vi "sortData.vi"(8 "error in (no error)":errorcluster, 9 "data":T1(array[cluster])=[[{"time"=0.0, "Channel"=refnum, "data"=0.8}, {"time"=29.998, "Channel"=refnum, "data"=0.0}], [{"time"=0.0, "Channel"=refnum, "data"=0.74}, {"time"=29.998, "Channel"=refnum, "data"=0.0}], [{"time"=29.998, "Channel"=refnum, "data"=0.8}, {"time"=33.5, "Channel"=refnum, "data"=0.0}]], 10 "times":dbl[](array[numeric]), 11 "ScriptEventList in":refnum<class "ScriptEventList.lvclass">) -> (0 "error out":errorcluster, 2 "data out":T1(array[cluster]), 3 "ScriptEventList out":refnum<class "ScriptEventList.lvclass">)   [LabVIEW 2011, in "Tools.lvlib" / "Scripting.lvlib" / "ScriptEventList.lvclass"]
uses:
  ScriptEventList.lvclass
  DatabaseHelpers/Database Objects/Channel/Channel.lvclass
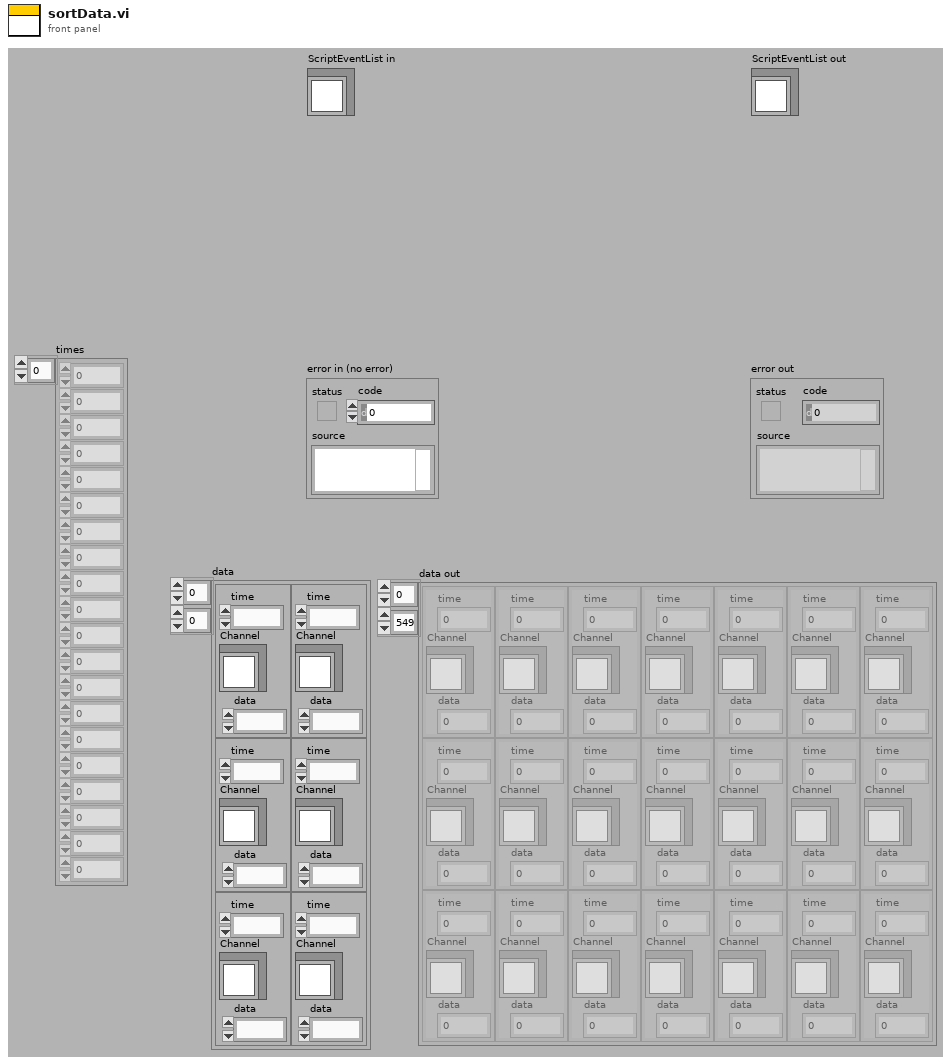
[diagram p1: front panel]
types:
  T1 = cluster{"time":dbl, "Channel":refnum<class "Channel.lvclass">, "data":dbl}[][]
  T2 = cluster{"time":dbl, "Channel":refnum<class "Channel.lvclass">, "data":dbl}[]
  T3 = cluster{"time":dbl, "Channel":refnum<class "Channel.lvclass">, "data":dbl}
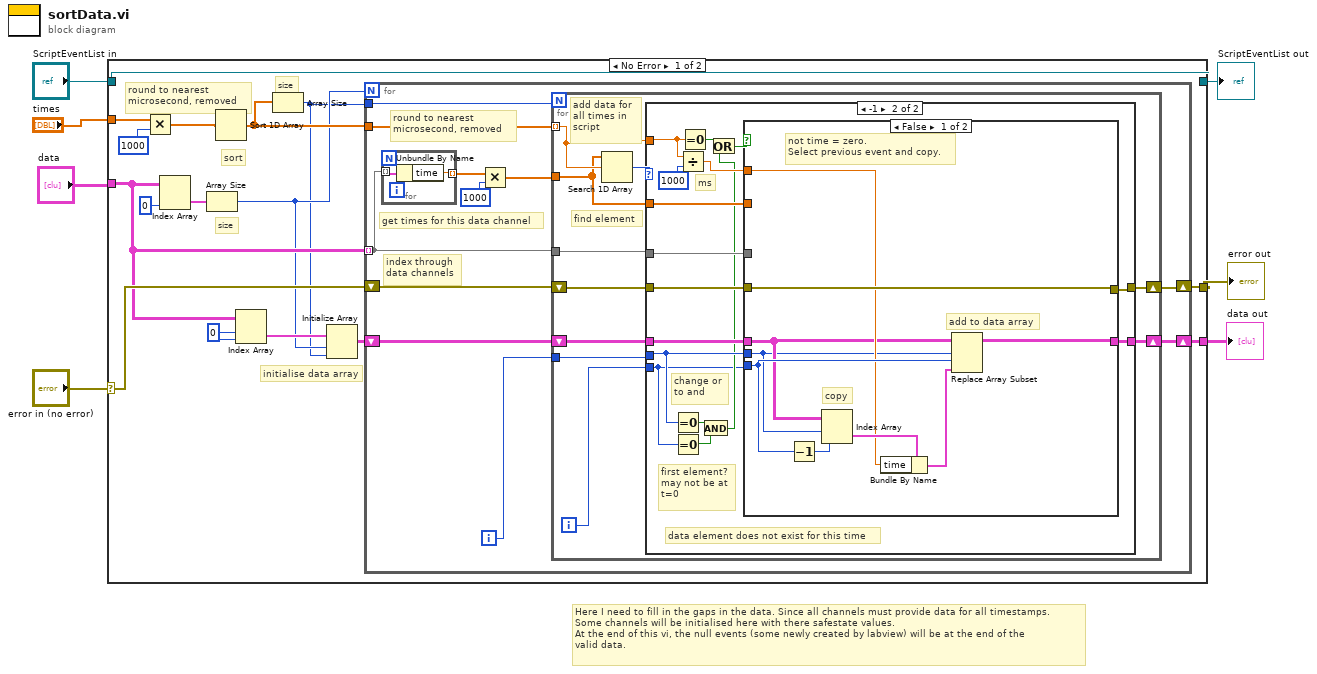
[diagram p0: block diagram]
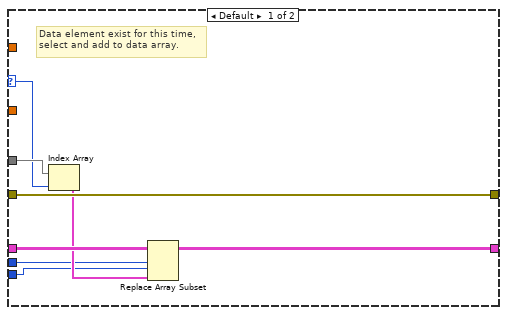
[diagram p2: hidden frame]
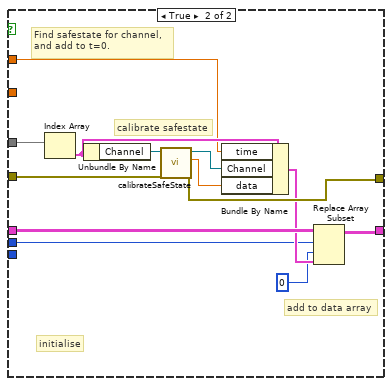
[diagram p3: hidden frame]
diagram:
  # "Here I need to fill in the gaps in the data. Since all channels must provide data for all timestamps.\nSome channels will be initialised here with there safestate values. \nAt the end of this vi, the null events (some newly created by labview) will be at the end of the \nvalid data."
  n1 = case shown="No Error" "error in (no error)" {
    selector: "error in (no error)" -> [w23 w94]
    tunnel: [w21 w94] -> w6
    tunnel: [w22 w93] -> w4
    tunnel: "ScriptEventList in" -> [w22 w93]
    tunnel: "times" -> [w10 _]
    tunnel: "data" -> [w19 _]
    tunnel: [w11 _] -> w1
    frame No Error {
      w17 = 0
      # "size"
      # "sort"
      # "round to nearest\nmicrosecond, removed"
      # "initialise data array"
      # "size"
      n2 = Multiply(x=w10, y=1000) -> (x*y=w8:dbl[])
      n3 = Index Array(array=w19, index (col)=0) -> (element=w15:T2)  [unwired: 1 in]
      n4 = Array Size(array=w15) -> (size(s)=w14:i32)
      n5 = Sort 1D Array(array=w8) -> (sorted array=w16:dbl[])
      n6 = Index Array(array=w19, index (row)=w17, index (col)=w17) -> (element=w18:T3)
      n7 = Array Size(array=w16) -> (size(s)=w13:i32)
      n8 = Initialize Array(w18, w14, w13) -> (w12:T1)
      n9 = for {
        N: w14 -> [_]
        tunnel: w16 -> [w32]
        shift-right: [w34] -> w21
        shift-left: w23 -> [w33]
        tunnel: w19 -> [w27] mode=indexing
        tunnel: w13 -> [w31]
        shift-right: [w28] -> w11
        shift-left: w12 -> [w30]
        i -> [w29]
        # "index through\ndata channels"
        # "get times for this data channel"
        # "round to nearest\nmicrosecond, removed"
        n10 = for {
          tunnel: w27 -> [w35] mode=indexing
          tunnel: [w36] -> w25 mode=indexing
          n11 = Unbundle By Name(w35) -> ("time"=w36:dbl)
        }
        n12 = Multiply(x=w25, y=1000) -> (x*y=w24:dbl[])
        n13 = for {
          N: w31 -> [_]
          shift-right: [w44] -> w34
          shift-left: w33 -> [w45]
          tunnel: w32 -> [w42] mode=indexing
          shift-right: [w38] -> w28
          shift-left: w30 -> [w41]
          tunnel: w29 -> [w40]
          tunnel: w24 -> [w37]
          tunnel: w27 -> [w43]
          i -> [w39]
          # "add data for \nall times in\nscript"
          # "find element"
          n14 = Search 1D Array(1D array=w37, element=w42) -> (index of element=w46:i32)  [unwired: 1 in]
          n15 = case shown="-1" w46 {
            selector: w46 -> [w48 _]
            tunnel: w42 -> [_ w64]
            tunnel: w37 -> [_ w70]
            tunnel: w43 -> [w51 w69]
            tunnel: w45 -> [w54 w68]
            tunnel: [w54 w67] -> w44
            tunnel: w39 -> [w47 w55]
            tunnel: w41 -> [w53 w66]
            tunnel: w40 -> [w49 w61]
            tunnel: [w52 w65] -> w38
            frame Default {
              # "Data element exist for this time,\nselect and add to data array."
              n16 = Index Array(array=w51, index=w48) -> (element=w50:T3)
              n17 = Replace Array Subset(array=w53, new element=w50, index (row)=w49, index (col)=w47) -> (w52:T1)
            }
            frame -1 {
              # "change or\nto and"
              # "first element?\nmay not be at\nt=0"
              # "ms"
              # "data element does not exist for this time"
              n18 = Equal To 0?(x=w61) -> (x = 0?=w58:bool)
              n19 = Equal To 0?(x=w55) -> (x = 0?=w56:bool)
              n20 = Divide(x=w64, y=1000) -> (x/y=w63:dbl)
              n21 = Equal To 0?(x=w64) -> (x = 0?=w60:bool)
              n22 = And(x=w58, y=w56) -> (x .and. y?=w57:bool)
              n23 = Or(x=w60, y=w57) -> (x .or. y?=w59:bool)
              n24 = case shown="False" w59 {
                tunnel: w63 -> [w75 w89]
                tunnel: w70 -> [_ _]
                tunnel: w69 -> [_ w80]
                tunnel: w68 -> [w79 w91]
                tunnel: [w79 w87] -> w67
                tunnel: w55 -> [w77 _]
                tunnel: w66 -> [w73 w85]
                tunnel: w61 -> [w71 w81]
                tunnel: [w78 w83] -> w65
                frame False {
                  # "add to data array"
                  # "copy"
                  # "not time = zero.\nSelect previous event and copy."
                  n25 = Decrement(x=w77) -> (x-1=w72:i32)
                  n26 = Index Array(array=w73, index (row)=w71, index (col)=w72) -> (element=w76:T3)
                  n27 = Bundle By Name(cluster=w76, "time"=w75) -> (w74:T3)
                  n28 = Replace Array Subset(array=w73, new element=w74, index (row)=w71, index (col)=w77) -> (w78:T1)
                }
                frame True {
                  # "add to data array"
                  # "calibrate safestate"
                  # "Find safestate for channel,\nand add to t=0."
                  # "initialise"
                  n29 = Index Array(array=w80) -> (element=w90:T3)  [unwired: 1 in]
                  n30 = Unbundle By Name(w90) -> ("Channel"=w92:refnum<class "Channel.lvclass">)
                  n31 = call "calibrateSafeState.vi"("error in (no error)"=w91, "Channel in"=w92) -> ("error out"=w87:errorcluster, "calibratedValue"=w86:dbl, "Channel out"=w88:refnum<class "Channel.lvclass">)  [unwired: 7 in]
                  n32 = Bundle By Name(cluster=w90, "time"=w89, "Channel"=w88, "data"=w86) -> (w84:T3)
                  n33 = Replace Array Subset(array=w85, new element=w84, index (row)=w81, index (col)=0) -> (w83:T1)
                }
              }
            }
          }
        }
      }
    }
    frame Error {
    }
  }
  "error out" <- w6
  "ScriptEventList out" <- w4
  "data out" <- w1
